vi "CryoCooler Generate HK List.vi"() -> (2 "Channel Names":string[](array[string])=["Telescope RA", "Telescope DEC", "Telescope Moving?", "Telescope Status"], 3 "Channel List":refnum<class "HK Item.lvclass">[](array[class]))   [LabVIEW 2024]
uses:
  hk-channel-class/hk-channel-class/HK Item/HK Item.lvclass
  hk-channel-class/hk-channel-class/HK Item/HK Channel Units and Setup.ctl
  hk-channel-class/hk-channel-class/HK Item/HK Channel enum Data Type.ctl
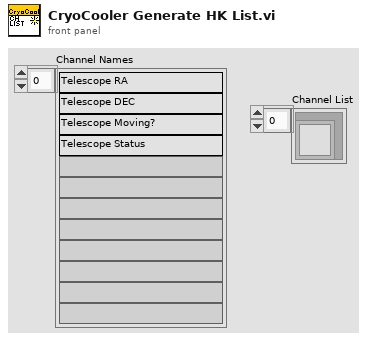
[diagram p1: front panel]
types:
  T1 = typedef "HK Item.lvclass/HK Channel Units and Setup.ctl" = cluster{"Unit Type":string, "Units":string, "Configuration":string, "Digits":i32, "Data Type":T2, "Exponential?":bool, "Source":string}
  T2 = typedef "HK Item.lvclass/HK Channel enum Data Type.ctl" = enum16{"Floating Point", "Integer", "Enum", "String", "Waveform", "File"}
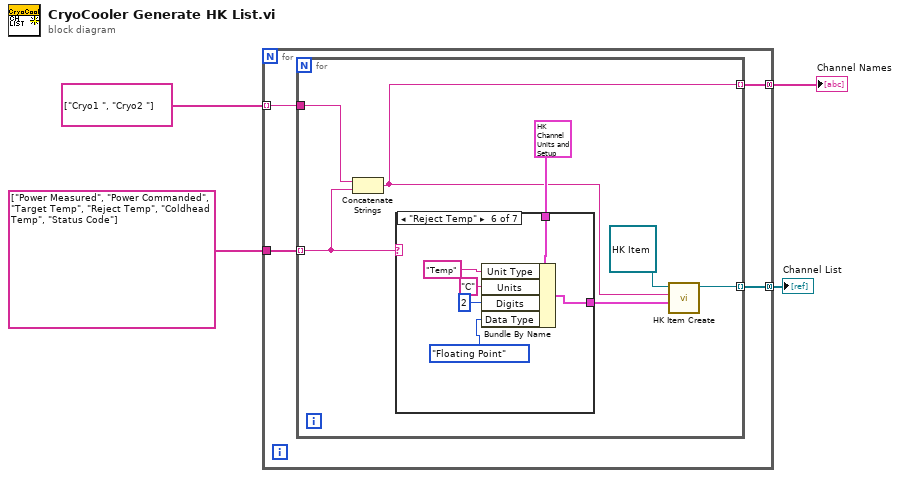
[diagram p0: block diagram]
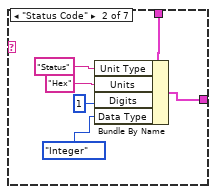
[diagram p3: hidden frame]
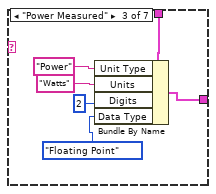
[diagram p4: hidden frame]
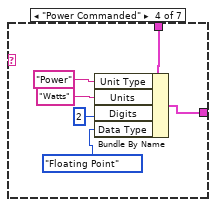
[diagram p5: hidden frame]
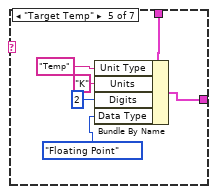
[diagram p6: hidden frame]
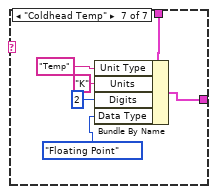
[diagram p7: hidden frame]
diagram:
  n1 = for {
    tunnel: string[] ["Power Measured", "Power Commanded", "Target Temp", "Reject Temp", "Coldhead Temp", "Status Code"] -> [w8]
    tunnel: [w7] -> w3 mode=concatenating
    tunnel: string[] ["Cryo1 ", "Cryo2 "] -> [w6] mode=indexing
    tunnel: [w5] -> w1 mode=concatenating
    n2 = for {
      tunnel: w8 -> [w10] mode=indexing
      tunnel: [w13] -> w7 mode=indexing
      tunnel: w6 -> [w11]
      tunnel: [w9] -> w5 mode=indexing
      n3 = Concatenate Strings(w11, w10) -> (w9:string)
      n4 = case shown="\"Reject Temp\"" w10 {
        tunnel: T1 {"Unit Type"="", "Units"="", "Configuration"="", "Digits"=3, "Data Type"=enum."Floating Point", "Exponential?"=FALSE, "Source"=""} ("Channel Setup") -> [w16 w22 w28 w34 w40 w46 w52]
        tunnel: [w16 w17 w23 w29 w36 w42 w48] -> w15
        frame "False", Default {
        }
        frame "Status Code" {
          n5 = Bundle By Name(cluster=w22, "Unit Type"="Status", "Units"="Hex", "Digits"=1, "Data Type"=HK_Channel_enum_Data_Type."Integer") -> (w17:T1)
        }
        frame "Power Measured" {
          n6 = Bundle By Name(cluster=w28, "Unit Type"="Power", "Units"="Watts", "Digits"=2, "Data Type"=HK_Channel_enum_Data_Type."Floating Point") -> (w23:T1)
        }
        frame "Power Commanded" {
          n7 = Bundle By Name(cluster=w34, "Unit Type"="Power", "Units"="Watts", "Digits"=2, "Data Type"=HK_Channel_enum_Data_Type."Floating Point") -> (w29:T1)
        }
        frame "Target Temp" {
          n8 = Bundle By Name(cluster=w40, "Unit Type"="Temp", "Units"="K", "Digits"=2, "Data Type"=HK_Channel_enum_Data_Type."Floating Point") -> (w36:T1)
        }
        frame "Reject Temp" {
          n9 = Bundle By Name(cluster=w46, "Unit Type"="Temp", "Units"="C", "Digits"=2, "Data Type"=HK_Channel_enum_Data_Type."Floating Point") -> (w42:T1)
        }
        frame "Coldhead Temp" {
          n10 = Bundle By Name(cluster=w52, "Unit Type"="Temp", "Units"="K", "Digits"=2, "Data Type"=HK_Channel_enum_Data_Type."Floating Point") -> (w48:T1)
        }
      }
      n11 = call-dynamic "HK Item Create.vi"("Channel Setup"=w15, "Name"=w9, "HK Item in"=refnum<class "HK Item.lvclass"> refnum) -> ("HK Item out"=w13:refnum<class "HK Item.lvclass">)  [unwired: 7 in, 1 out]
    }
  }
  "Channel List" <- w3
  "Channel Names" <- w1
